vi "Process.vi"(8 "error in":errorcluster, 11 "Logger":refnum<class "Logger.PGSQL.lvclass">) -> (0 "error out":errorcluster, 3 "Logger out":refnum<class "Logger.PGSQL.lvclass">)   [LabVIEW 2019, in "Logger.PGSQL.lvlib" / "Logger.PGSQL.lvclass"]
doc: "---------------------------------------------------------------\nJKI State Machine Objects™\nhttp://jki.net/state-machine-objects/\nCopyright (C) 2005-2015, JKI <info@jki.net>\nALL RIGHTS RESERVED"
uses:
  Logger.PGSQL.lvclass
  C:/Program Files (x86)/National Instruments/LabVIEW 2019/vi.lib/JKI/JKI SMO/SMO/SMO.lvclass
  Logger.PGSQL.lvclass/Logger.PGSQL.ctl
  <vilib>/JKI/JKI SMO/SMO/SMO.lvclass/SMO.ctl
  <vilib>/JKI/JKI SMO/SMO/Private/ReftoDVR--SMO.vi
  <userlib>/LevyLab/LV-Data/LV-Data.PG/Private/INSERT Multivalue.vi
  <userlib>/LevyLab/Logger/Logger/Logger.lvclass
  <userlib>/LevyLab/Debug/Debug.lvlib
  <vilib>/JKI/JKI SMO/SMO/SMO.lvclass
  C:/Program Files (x86)/National Instruments/LabVIEW 2019/user.lib/LevyLab/Logger/Logger/Logger.lvclass
panel:
  out "Status":string
  out "State History":string
  out "Status Log":string
  out "Data":variant
  out "Address(es)":string
  # "DB Logger"
  # "For instructions on how to use the JKI State Machine Objects, examples and video tutorials, visit:\nhttp://jki.net/state-machine-objects/\n\nJKI State Machine Objects™\nhttp://jki.net/state-machine-objects/\nCopyright (C) 2005-2015, JKI <info@jki.net>\nALL RIGHTS RESERVED"
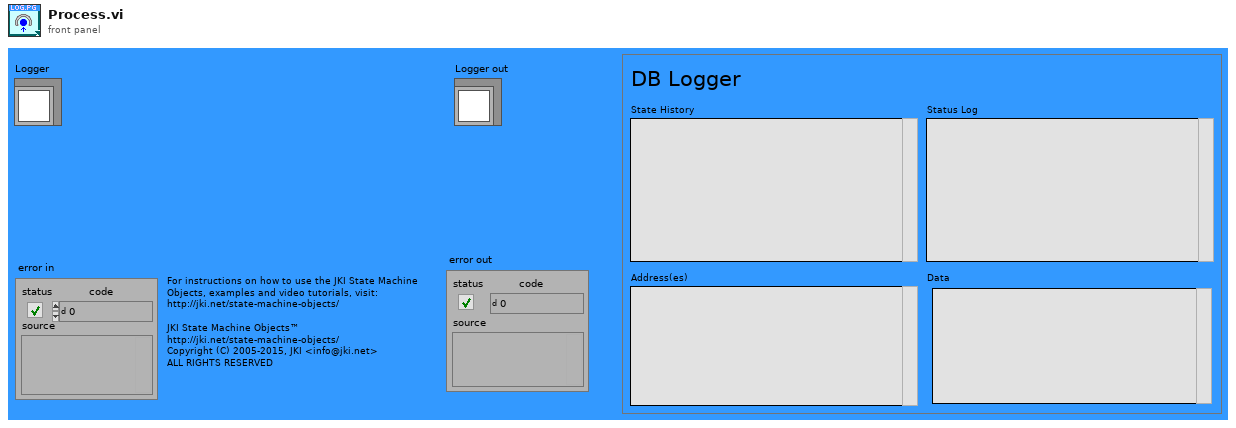
[diagram p1: front panel]
types:
  T1 = enum32{"invalid app kind", "Development System", "Run Time System", "Student Edition", "Embedded LabVIEW", "Evaluation", "Custom"}
  T2 = enum16{"unconfigured", "disconnected", "connected"}
  T3 = enum32{"Invalid", "Standard", "Closed", "Hidden", "Minimized", "Maximized"}
  T4 = cluster{"Core":cluster{"Current VI Reference":refnum<vi>, "Close Panel on Exit?":bool, "Last Error":cluster{"error":errorcluster, "previous state":string, "remaining states":string}, "Shutdown?":bool}, "SelfRef":refnum<class "Logger.PGSQL.lvclass">, "address":string, "data in":variant, "timestamps":timestamp[], "data out":variant, "Write Time":timestamp}
  T5 = cluster{"Current VI Reference":refnum<vi>, "Close Panel on Exit?":bool, "Last Error":cluster{"error":errorcluster, "previous state":string, "remaining states":string}, "Shutdown?":bool}
  T6 = typedef "Debug.lvlib/Attribute.Debug.lvclass/DebugBehavior.ctl" = enum16{"Normal", "Debug"}
  T7 = typedef "SMO.lvclass/Protected Events.ctl" = cluster{"StopProcesses":refnum<user-event>, "AbortProcesses":refnum<user-event>, "Config Changed":refnum<user-event>, "Dependency":refnum<user-event>}
  T8 = typedef "Logger.PGSQL.lvlib/Logger.PGSQL.lvclass/PrivateEvents--Cluster.ctl" = cluster{"Set Address":refnum<user-event>, "Write Variable":refnum<user-event>, "Read Variable":refnum<user-event>, "Write Variable Multiline":refnum<user-event>}
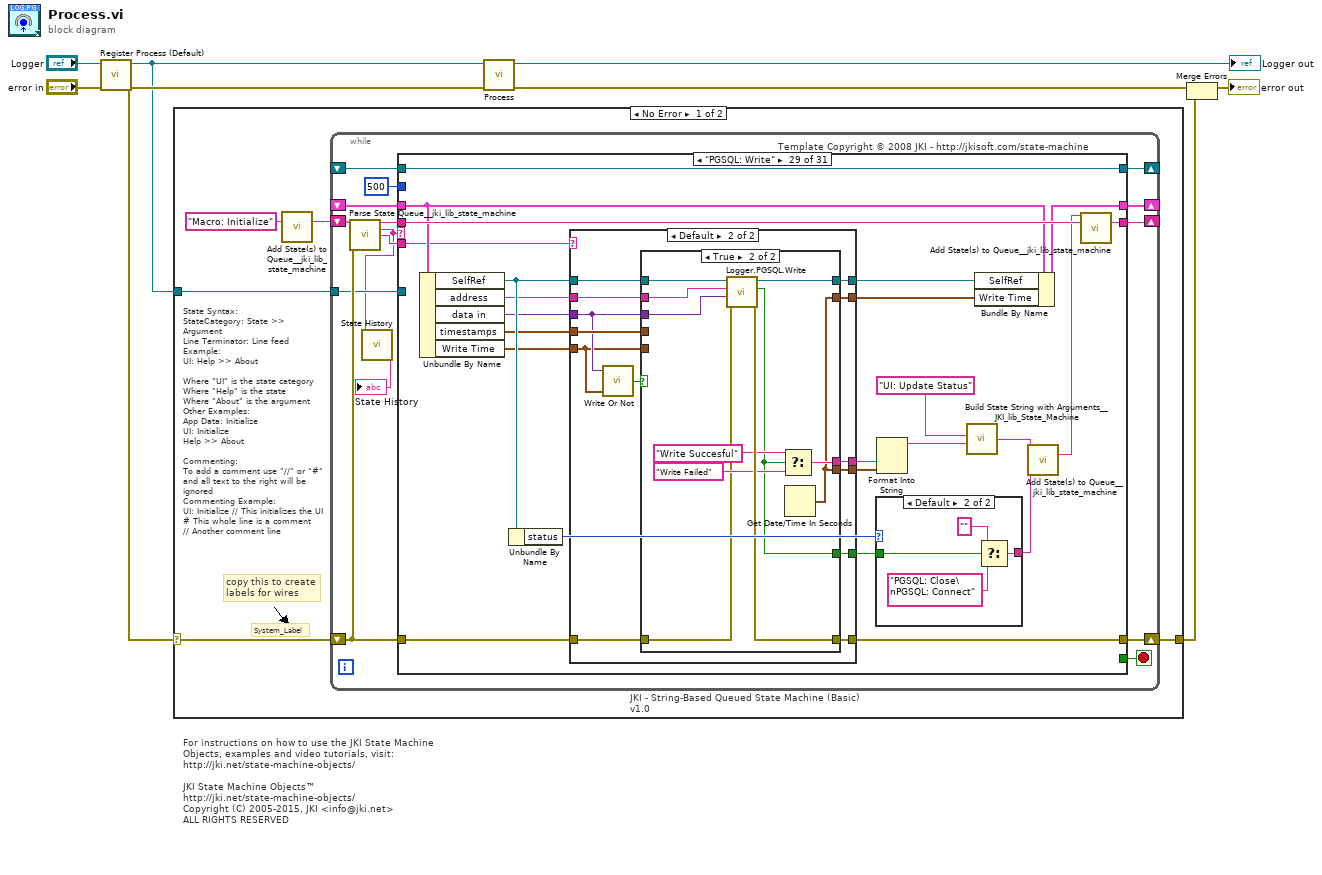
[diagram p0: block diagram]
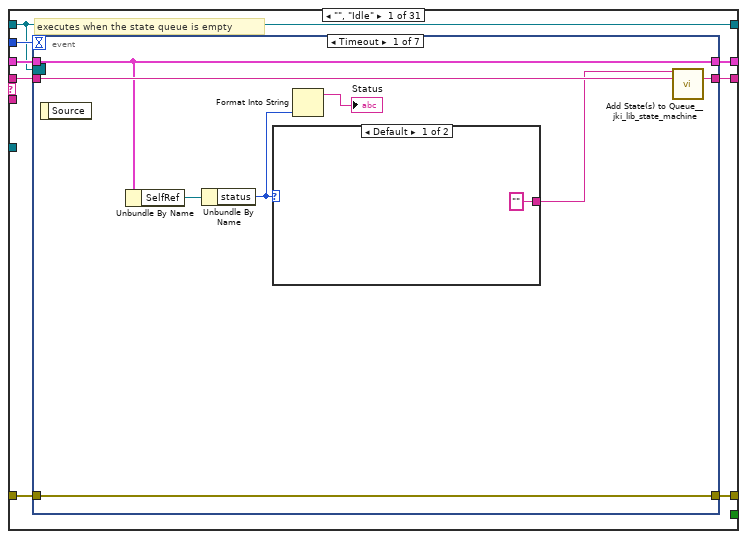
[diagram p2: hidden frame]
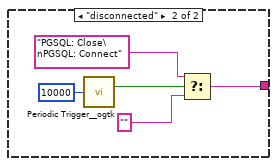
[diagram p3: hidden frame]
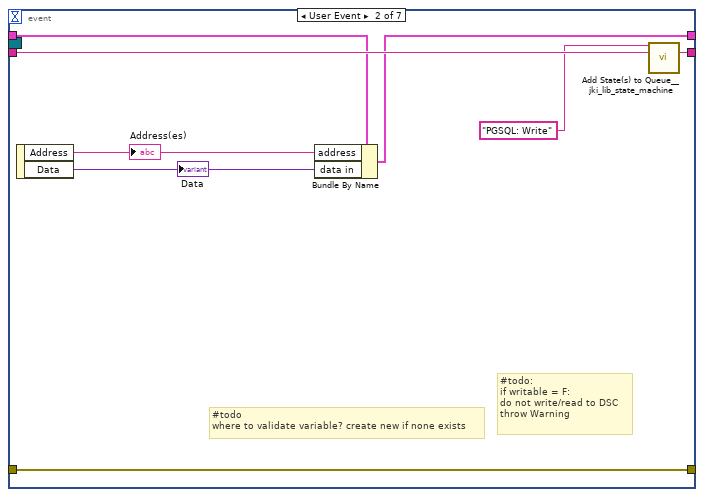
[diagram p4: hidden frame]
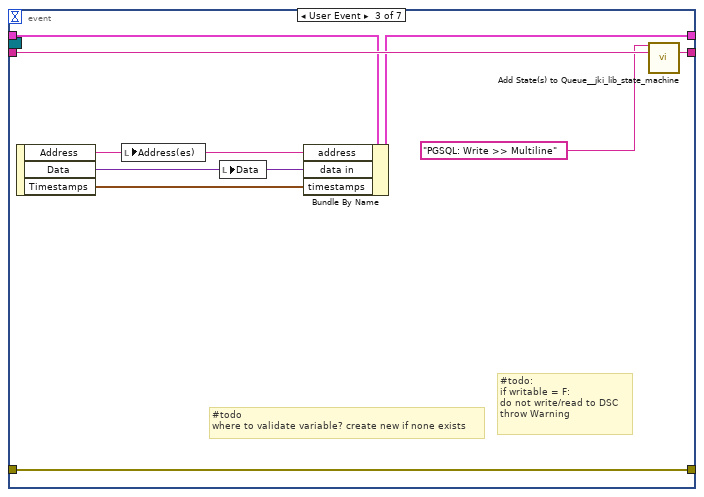
[diagram p5: hidden frame]
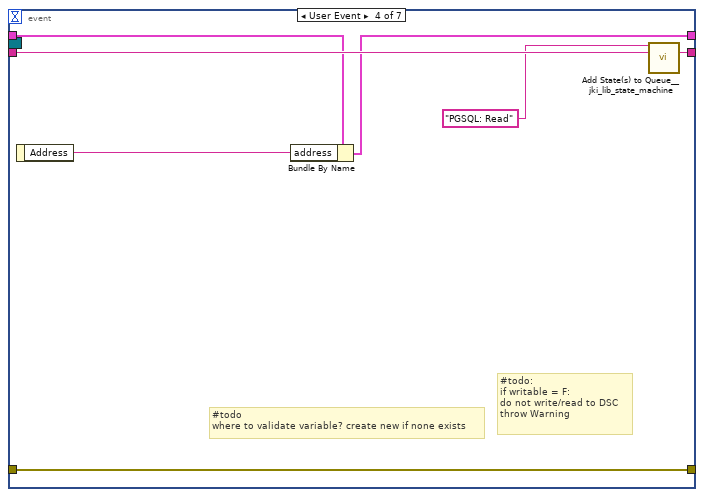
[diagram p6: hidden frame]
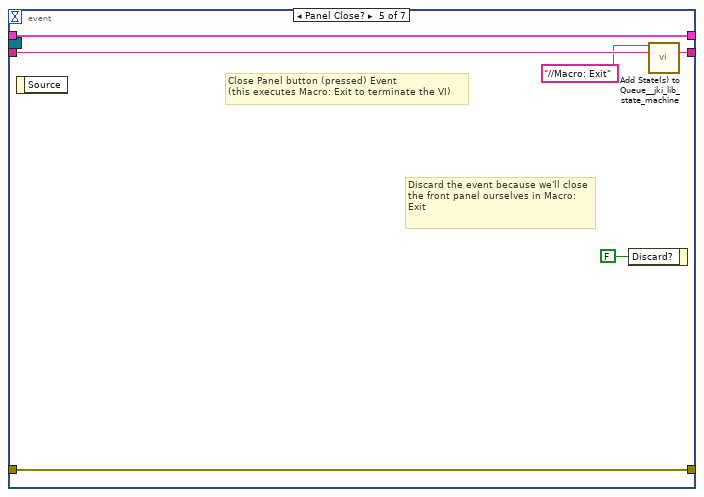
[diagram p7: hidden frame]
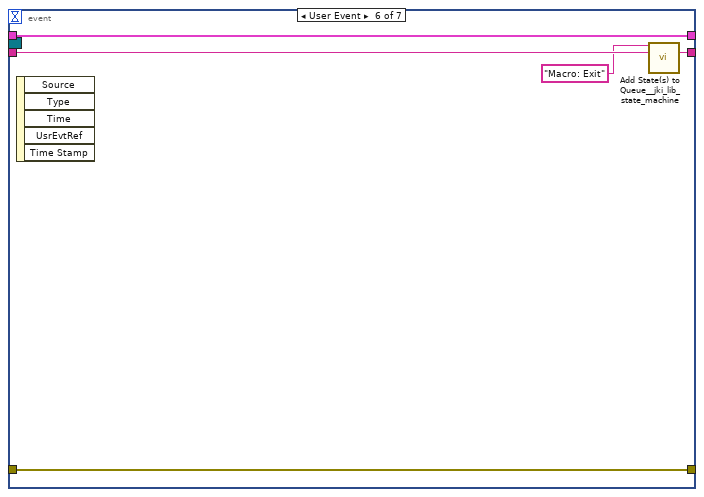
[diagram p8: hidden frame]
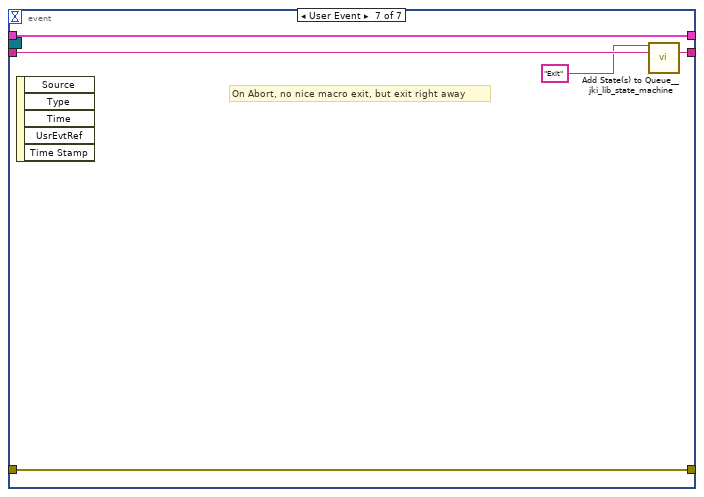
[diagram p9: hidden frame]
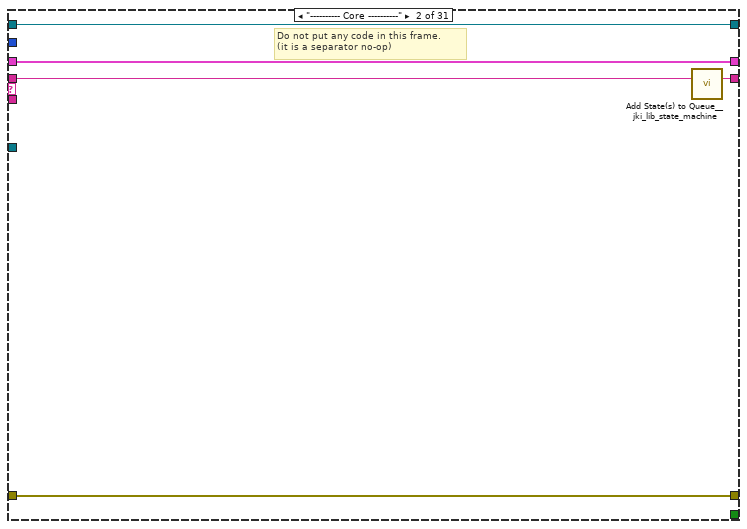
[diagram p10: hidden frame]
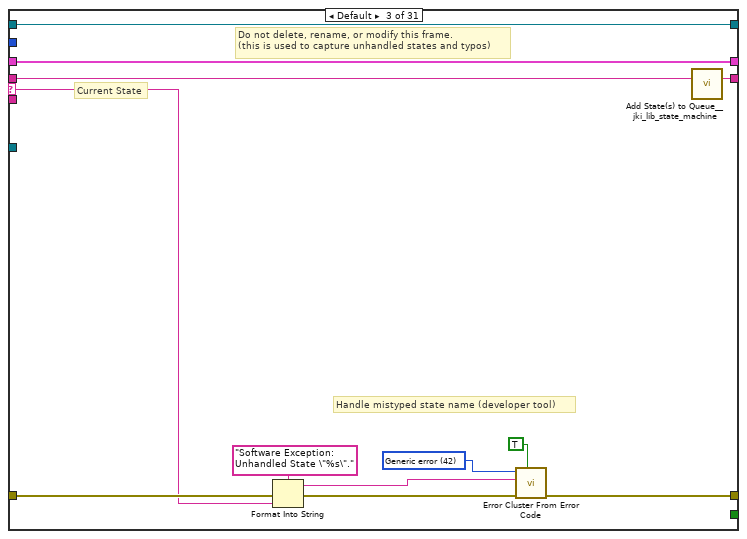
[diagram p11: hidden frame]
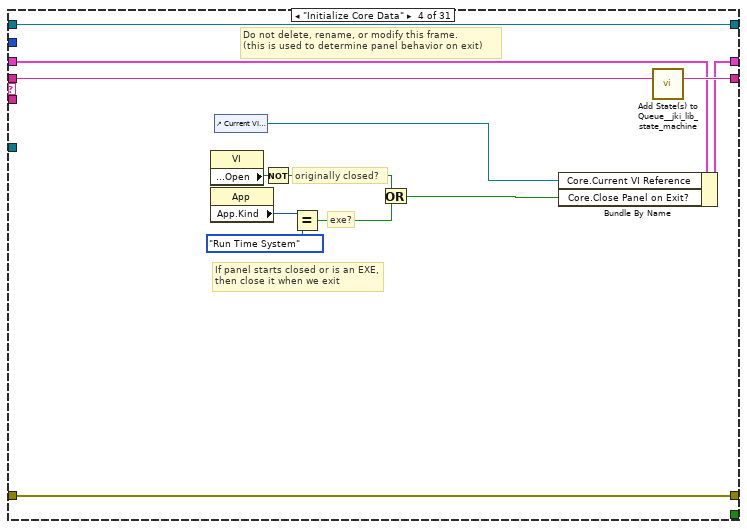
[diagram p12: hidden frame]
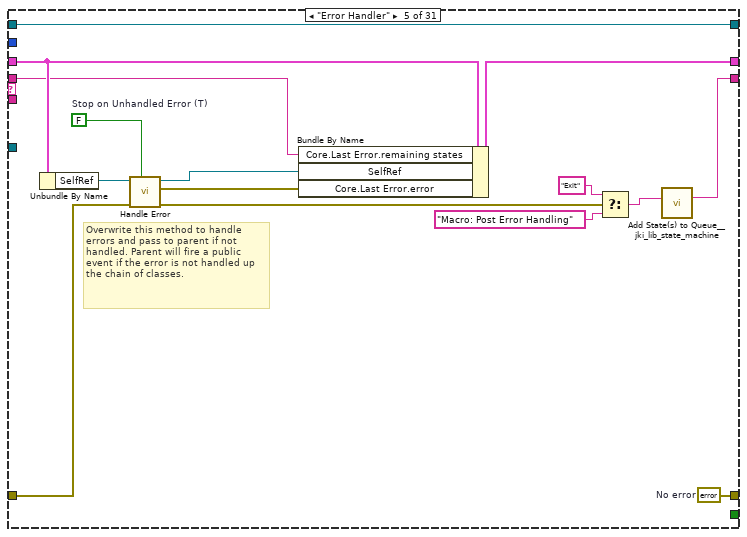
[diagram p13: hidden frame]
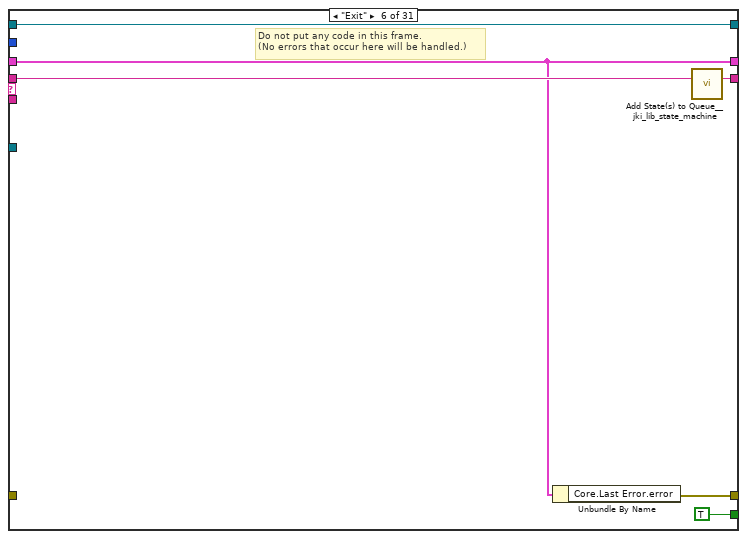
[diagram p14: hidden frame]
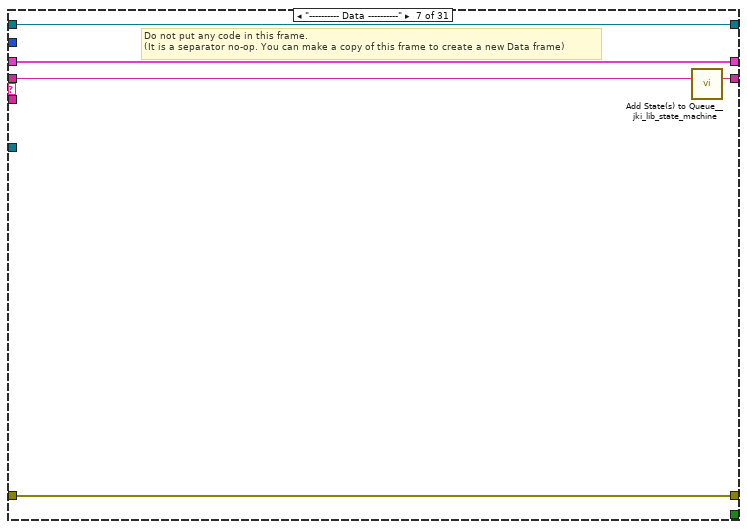
[diagram p15: hidden frame]
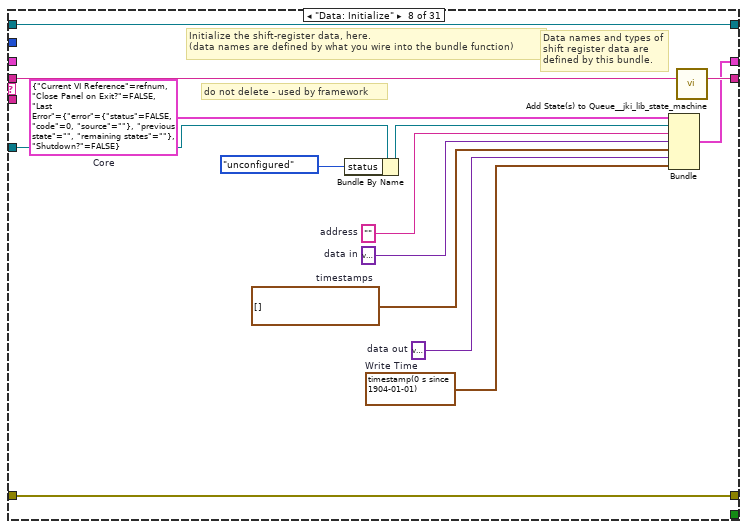
[diagram p16: hidden frame]
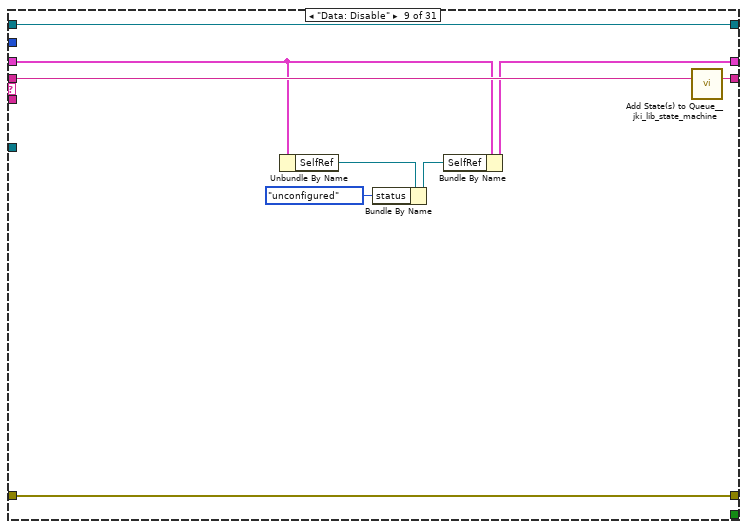
[diagram p17: hidden frame]
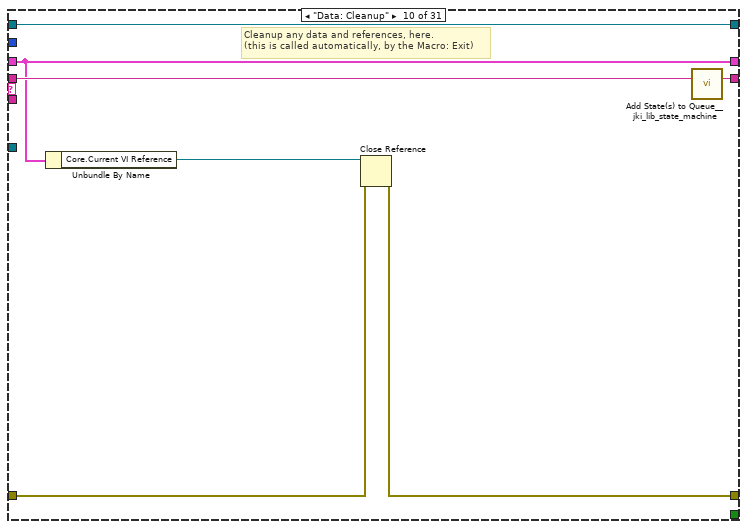
[diagram p18: hidden frame]
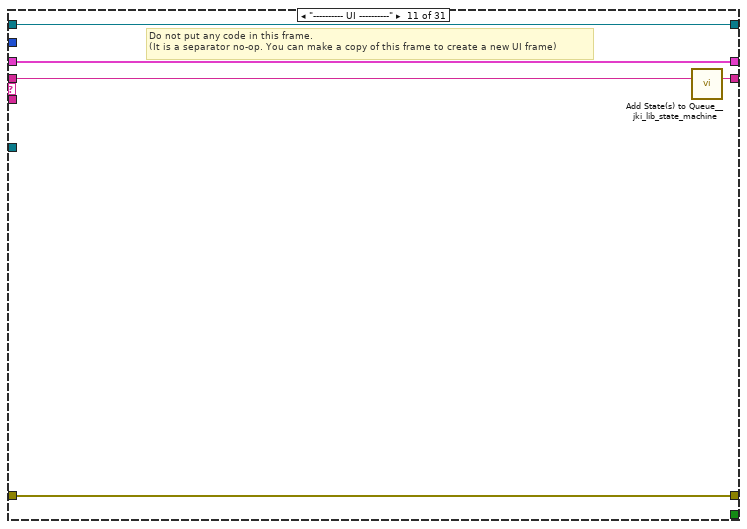
[diagram p19: hidden frame]
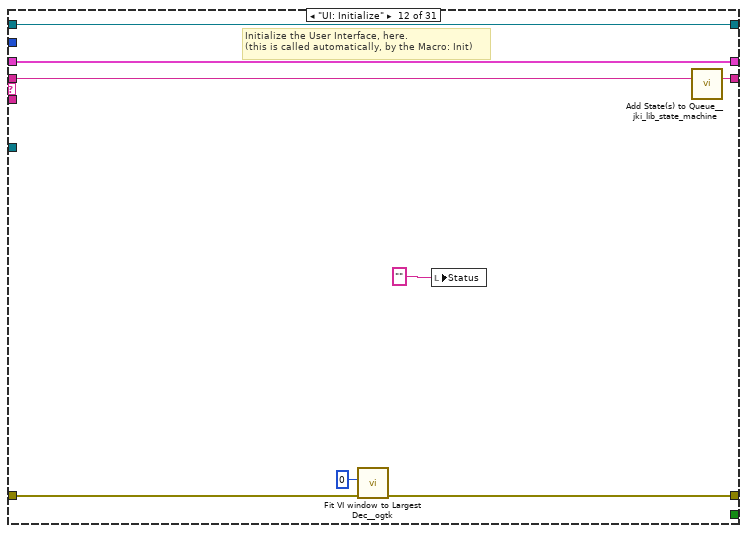
[diagram p20: hidden frame]
diagram:
  # "For instructions on how to use the JKI State Machine Objects, examples and video tutorials, visit:\nhttp://jki.net/state-machine-objects/\n\nJKI State Machine Objects™\nhttp://jki.net/state-machine-objects/\nCopyright (C) 2005-2015, JKI <info@jki.net>\nALL RIGHTS RESERVED"
  n1 = call <vilib>:"Register Process (Default).vi"("error in (no error)"="error in", "SMO"="Logger") -> ("error out"=w5:errorcluster, "SelfRef"=w4:refnum<class "Logger.PGSQL.lvclass">)  [unwired: 8 in]
  n2 = case shown="No Error" w5 {
    selector: w5 -> [w10 w477]
    tunnel: w4 -> [w11 _]
    tunnel: [w9 w477] -> w2
    frame No Error {
      # "State Syntax:\nStateCategory: State >> Argument\nLine Terminator: Line feed\nExample:\nUI: Help >> About\n\nWhere \"UI\" is the state category\nWhere \"Help\" is the state\nWhere \"About\" is the argument\nOther Examples:\nApp Data: Initialize\nUI: Initialize\nHelp >> About\n\nCommenting:\nTo add a comment use \"//\" or \"#\" and all text to the right will be ignored\nCommenting Example:\nUI: Initialize // This initializes the UI\n# This whole line is a comment\n// Another comment line"
      # "copy this to create labels for wires"
      # "System_Label"
      n3 = call <vilib>:"Add State(s) to Queue__jki_lib_state_machine.vi"("State(s) in (\"\")"="Macro: Initialize") -> ("States Out"=w13:string)  [unwired: 14 in]
      n4 = while "JKI - String-Based Queued State Machine (Basic) v1.0" {
        shift-right: [w23] -> _
        shift-left: _ -> [w22]
        shift-right: [w14] -> w9
        shift-left: w10 -> [w20]
        shift-right: [w25] -> _
        shift-left: w13 -> [w26]
        tunnel: w11 -> [w19]
        shift-right: [w18] -> _
        shift-left: _ -> [w17]
        stop <- w24 stop-if-true
        # "Template Copyright © 2008 JKI - http://jkisoft.com/state-machine"
        n5 = call <vilib>:"Parse State Queue__jki_lib_state_machine.vi"("State Queue"=w26, "Error In (no error)"=w20) -> ("Remaining States"=w28:string, "Current State"=w15:string, "Arguments"=w27:string)  [unwired: 11 in]
        n6 = call <userlib>:"State History.vi"("Current State"=w15) -> ("History"=→"State History":string)  [unwired: 10 in]
        n7 = case shown="\"PGSQL: Write\"" w15 {
          selector: w15 -> [_ _ w97 _ _ _ _ _ _ _ _ _ _ _ _ _ _ _ _ _ _ _ _ _ _ _ _ _ _ _ _]
          tunnel: w28 -> [w36 w95 w101 w120 w125 w141 w146 w160 w169 w176 w181 w189 w197 w204 w219 w227 w259 w270 w284 w302 w333 w338 w349 w354 w367 w373 w378 w387 w410 w467 w476]
          tunnel: w27 -> [_ _ _ _ _ _ _ _ _ _ _ _ w191 w198 w213 w221 _ _ _ _ _ _ _ _ _ _ _ _ w389 _ _]
          tunnel: w22 -> [w34 w92 w99 w111 w131 w137 w143 _ w164 w171 w178 w187 w194 w202 w216 w223 w256 w264 w272 w292 w318 w335 w346 w351 w365 w371 w376 w383 w406 w464 w473]
          tunnel: w20 -> [w32 w93 w102 w117 w133 _ w144 w151 w166 w173 w179 w184 w195 w200 w217 w225 w257 w260 w282 w300 w331 w336 w341 w352 w361 w369 w374 w380 w404 w462 w469]
          tunnel: [w35 w94 w100 w119 w123 w140 w145 w159 w168 w175 w180 w188 w196 w203 w218 w226 w258 w269 w283 w301 w332 w337 w348 w353 w366 w372 w377 w386 w409 w466 w475] -> w25
          tunnel: [_ _ _ _ _ TRUE _ _ _ _ _ _ _ _ _ _ _ _ _ _ _ _ _ _ _ _ _ _ _ _ _] -> w24
          tunnel: [w31 w92 w99 w118 w130 w137 w143 w158 w165 w171 w178 w187 w194 w202 w216 w223 w256 w264 w273 w293 w319 w335 w346 w351 w365 w371 w376 w384 w405 w464 w472] -> w23
          tunnel: 500 ("Timeout") -> [w30 _ _ _ _ _ _ _ _ _ _ _ _ _ _ _ _ _ _ _ _ _ _ _ _ _ _ _ _ _ _]
          tunnel: w19 -> [_ _ _ _ _ _ _ w148 _ _ _ _ _ _ _ _ _ _ _ _ _ _ _ _ _ _ _ _ _ _ _]
          tunnel: [w29 w91 w96 w108 w135 w138 w142 w157 w167 w170 w177 w186 w193 w201 w215 w220 w255 w268 w281 w299 w326 w334 w347 w350 w364 w370 w375 w385 w408 w465 w474] -> w18
          tunnel: w17 -> [w29 w91 w96 w108 w135 w138 w142 w157 w167 w170 w177 w186 w193 w201 w215 w220 w255 w268 w281 w299 w326 w334 w347 w350 _ w370 w375 w385 w408 w465 w474]
          tunnel: [w33 w93 w103 w117 w132 w136 w144 w151 w166 w172 w179 w185 w195 w199 w217 w224 w257 w260 w282 w300 w331 w336 w340 w352 w360 w369 w374 w379 w407 w461 w468] -> w14
          frame "", "Idle" {
            # "executes when the state queue is empty"
            n8 = event shown="[0] Timeout" {
              selector: w29 -> [_ _ _ _ _ _ _]
              dyn-events: _ -> [_ _ _ _ _ _ _]
              timeout: w30 -> [_ _ _ _ _ _ _]
              tunnel: w36 -> [w44 w58 w67 w74 w80 w85 w90]
              tunnel: [w43 w57 w66 w73 w79 w84 w89] -> w35
              tunnel: w34 -> [w41 w55 w64 w71 w77 w82 w87]
              tunnel: [w42 w56 w65 w72 w78 w83 w88] -> w33
              tunnel: w32 -> [w42 w56 w65 w72 w78 w83 w88]
              tunnel: [w41 w52 w60 w69 w77 w82 w87] -> w31
              event Timeout {
                n9 = event-data() -> ()  [unwired: 1 in, 1 out]
                n10 = Unbundle By Name(w41) -> ("SelfRef"=w40:refnum<class "Logger.PGSQL.lvclass">)
                n11 = Unbundle By Name(w40) -> ("status"=w38:T2)
                n12 = case shown="Default" w38 {
                  tunnel: ["" w48] -> w39
                  frame Default {
                  }
                  frame "disconnected" {
                    n13 = call <userlib>:"Periodic Trigger__ogtk.vi"("time (ms)"=u32 10000) -> ("Triggered"=w50:bool)  [unwired: 12 in, 2 out]
                    n14 = Select(t="PGSQL: Close\nPGSQL: Connect", s=w50, f="") -> (s? t:f=w48:string)
                  }
                }
                n15 = Format Into String(w38) -> (resulting string=→"Status":string)  [unwired: 3 in, 1 out]
                n16 = call <vilib>:"Add State(s) to Queue__jki_lib_state_machine.vi"("State(s) in Front (\"\")"=w39, "State(s) in (\"\")"=w44) -> ("States Out"=w43:string)  [unwired: 13 in]
              }
              event User Event {
                # "#todo:\nif writable = F:\ndo not write/read to DSC\nthrow Warning"
                # "#todo\nwhere to validate variable? create new if none exists"
                n17 = event-data() -> ("Address"=w53:string, "Data"=w54:variant)  [unwired: 1 in]
                "Address(es)" <- w53
                "Data" <- w54
                n18 = Bundle By Name(cluster=w55, "address"=w53, "data in"=w54) -> (w52:T4)
                n19 = call <vilib>:"Add State(s) to Queue__jki_lib_state_machine.vi"("State(s) in Front (\"\")"="PGSQL: Write" ("State(s) in Front (\"\")"), "State(s) in (\"\")"=w58) -> ("States Out"=w57:string)  [unwired: 13 in]
              }
              event User Event {
                # "#todo:\nif writable = F:\ndo not write/read to DSC\nthrow Warning"
                # "#todo\nwhere to validate variable? create new if none exists"
                n20 = event-data() -> ("Address"=w63:string, "Data"=w62:variant, "Timestamps"=w61:timestamp[])  [unwired: 1 in]
                n21 = local write "Address(es)"(w63) -> ()
                n22 = local write "Data"(w62) -> ()
                n23 = Bundle By Name(cluster=w64, "address"=w63, "data in"=w62, "timestamps"=w61) -> (w60:T4)
                n24 = call <vilib>:"Add State(s) to Queue__jki_lib_state_machine.vi"("State(s) in Front (\"\")"="PGSQL: Write >> Multiline" ("State(s) in Front (\"\")"), "State(s) in (\"\")"=w67) -> ("States Out"=w66:string)  [unwired: 13 in]
              }
              event User Event {
                # "#todo:\nif writable = F:\ndo not write/read to DSC\nthrow Warning"
                # "#todo\nwhere to validate variable? create new if none exists"
                n25 = event-data() -> ("Address"=w70:string)  [unwired: 1 in]
                n26 = Bundle By Name(cluster=w71, "address"=w70) -> (w69:T4)
                n27 = call <vilib>:"Add State(s) to Queue__jki_lib_state_machine.vi"("State(s) in Front (\"\")"="PGSQL: Read" ("State(s) in Front (\"\")"), "State(s) in (\"\")"=w74) -> ("States Out"=w73:string)  [unwired: 13 in]
              }
              event Panel Close? {
                # "Discard the event because we'll close the front panel ourselves in Macro: Exit"
                # "Close Panel button (pressed) Event\n(this executes Macro: Exit to terminate the VI)"
                n28 = event-data() -> ()  [unwired: 1 in, 1 out]
                n29 = event-data("Discard?"=FALSE) -> ()  [unwired: 1 in, 1 out]
                n30 = call <vilib>:"Add State(s) to Queue__jki_lib_state_machine.vi"("State(s) in Front (\"\")"="//Macro: Exit", "State(s) in (\"\")"=w80) -> ("States Out"=w79:string)  [unwired: 13 in]
              }
              event User Event {
                n31 = event-data() -> ()  [unwired: 1 in, 5 out]
                n32 = call <vilib>:"Add State(s) to Queue__jki_lib_state_machine.vi"("State(s) in Front (\"\")"="Macro: Exit", "State(s) in (\"\")"=w85) -> ("States Out"=w84:string)  [unwired: 13 in]
              }
              event User Event {
                # "On Abort, no nice macro exit, but exit right away"
                n33 = event-data() -> ()  [unwired: 1 in, 5 out]
                n34 = call <vilib>:"Add State(s) to Queue__jki_lib_state_machine.vi"("State(s) in Front (\"\")"="Exit", "State(s) in (\"\")"=w90) -> ("States Out"=w89:string)  [unwired: 13 in]
              }
            }
          }
          frame "---------- Core ----------" {
            # "Do not put any code in this frame.\n(it is a separator no-op)"
            n35 = call <vilib>:"Add State(s) to Queue__jki_lib_state_machine.vi"("State(s) in (\"\")"=w95) -> ("States Out"=w94:string)  [unwired: 14 in]
          }
          frame Default {
            w106 = 42 items=["No error", "Argument error", "Memory is full", "Out of zone", "End of file", "File already open", "Generic file I/O error", "File not found", "File permission error", "Disk is full", "Duplicate path", "Too many files open", "System feature not enabled", "Resource file not found", "Cannot add resource", "Resource not found", "Image not found", "Image memory error", "Pen does not exist", "Config type invalid", "Config token not found", "Config parse error", "Config memory error", "Bad external code format", "Bad external code offset", "External code not present", "Null window", "Destroy window error", "Null menu", "Print aborted", "Bad print record", "Print driver error", "Windows error during printing", "Memory error during printing", "Print dialog error", "Generic print error", "Invalid device refnum", "Device not found", "Device parameter error", "Device unit error", "Cannot open device", "Device call aborted", "Generic error", "Cancelled by user", "Object ID too low", "Object ID too high", "Object not in heap", "Unknown heap", "Unknown object (invalid DefProc)", "Unknown object (DefProc not in table)", "Message out of range", "Invalid (null) method", "Unknown message", "Manager call not supported", "Bad address", "Network operation in progress", "Network operation timed out", "Connection is busy", "Network attribute not supported", "Network error", "Address in use", "System out of memory", "Connection aborted", "Connection refused", "Not connected", "Already connected", "Connection closed", "Initialization error (interapplication manager)", "Bad occurrence", "Wait on unbound occurrence handler", "Occurrence queue overflow", "Datalog type conflict", "Unused", "Unrecognized type (interapplication manager)", "Memory corrupt", "Failed to make temporary DLL", "Old CIN version", "Drag socket not found", "Failed to load drop-object", "Failed to register OLE object", "Failed to release OLE object", "Format specifier type mismatch", "Unknown format specifier", "Too few format specifiers", "Too many format specifiers", "Scan failed", "Newer CIN version", "Error converting to variant", "Runtime menu error", "Password tampered", "Variant attribute not found", "Incompatible variant data type", "Event data is not available", "Event Store is not present", "Occurrence is not found", "Event Queue is not created", "Event info is not available", "Refnum passed is NULL", "Error retrieving Class GUID", "Error retrieving CoClass GUID", "Error retrieving TypeLib GUID.", "Bad built application magic bytes.", "Specific driver is different from the specific driver associated with the Logical Name.", "There is no session opened to the class driver.", "Max Error", "MAX - Error with config objects", "MAX - Error loading configuration", "MAX - Group not supported"]
            # "Current State"
            # "Do not delete, rename, or modify this frame.\n(this is used to capture unhandled states and typos)"
            # "Handle mistyped state name (developer tool)"
            n36 = Format Into String(format string="Software Exception: Unhandled State \"%s\"." ("message"), error in=w102, w97) -> (resulting string=w105:string, error out=w104:errorcluster)  [unwired: 1 in]
            n37 = call <vilib>:"Error Cluster From Error Code.vi"("show call chain? (False)"=TRUE, "error in (no error)"=w104, "error message (\"\")"=w105, "error code (0)"=w106) -> ("error out"=w103:errorcluster)  [unwired: 5 in]
            n38 = call <vilib>:"Add State(s) to Queue__jki_lib_state_machine.vi"("State(s) in (\"\")"=w101) -> ("States Out"=w100:string)  [unwired: 14 in]
          }
          frame "Initialize Core Data" {
            # "Do not delete, rename, or modify this frame.\n(this is used to determine panel behavior on exit)"
            # "originally closed?"
            # "exe?"
            # "If panel starts closed or is an EXE, then close it when we exit"
            n39 = property class="VI"() -> ("Front Panel.Open"=w116:bool)  [unwired: 2 in, 2 out]
            n40 = property class="App"() -> ("App.Kind"=w115:T1)  [unwired: 2 in, 2 out]
            n41 = control-ref of="Current VI Reference"() -> (w109:refnum<vi>)
            n42 = Not(x=w116) -> (.not. x?=w113:bool)
            n43 = Equal?(x=w115, y=T1."Run Time System" ("Application:Kind")) -> (x = y?=w112:bool)
            n44 = Or(x=w113, y=w112) -> (x .or. y?=w110:bool)
            n45 = Bundle By Name(cluster=w111, "Core.Current VI Reference"=w109, "Core.Close Panel on Exit?"=w110) -> (w118:T4)
            n46 = call <vilib>:"Add State(s) to Queue__jki_lib_state_machine.vi"("State(s) in (\"\")"=w120) -> ("States Out"=w119:string)  [unwired: 14 in]
          }
          frame "Error Handler" {
            w127 = FALSE  # Stop on Unhandled Error (T)
            w132 = errorcluster {"status"=FALSE, "code"=0, "source"=""}  # No error
            # "Overwrite this method to handle errors and pass to parent if not handled. Parent will fire a public event if the error is not handled up the chain of classes."
            n47 = Unbundle By Name(w131) -> ("SelfRef"=w134:refnum<class "Logger.PGSQL.lvclass">)
            n48 = call-dynamic "Handle Error.vi"("Stop on Unhandled Error (T)"=w127, "error in"=w133, "Logger.PGSQL"=w134) -> ("handling error"=w128:errorcluster, "Unhandled error"=w126:errorcluster, "Logger.PGSQL out"=w121:refnum<class "Logger.PGSQL.lvclass">)  [unwired: 6 in]
            n49 = Bundle By Name(cluster=w131, "Core.Last Error.remaining states"=w125, "SelfRef"=w121, "Core.Last Error.error"=w126) -> (w130:T4)
            n50 = Select(t="Exit", s=w128, f="Macro: Post Error Handling") -> (s? t:f=w122:string)
            n51 = call <vilib>:"Add State(s) to Queue__jki_lib_state_machine.vi"("State(s) in (\"\")"=w122) -> ("States Out"=w123:string)  [unwired: 14 in]
          }
          frame "Exit" {
            # "Do not put any code in this frame.\n(No errors that occur here will be handled.)"
            n52 = Unbundle By Name(w137) -> ("Core.Last Error.error"=w136:errorcluster)
            n53 = call <vilib>:"Add State(s) to Queue__jki_lib_state_machine.vi"("State(s) in (\"\")"=w141) -> ("States Out"=w140:string)  [unwired: 14 in]
          }
          frame "---------- Data ----------" {
            # "Do not put any code in this frame.\n(It is a separator no-op. You can make a copy of this frame to create a new Data frame)"
            n54 = call <vilib>:"Add State(s) to Queue__jki_lib_state_machine.vi"("State(s) in (\"\")"=w146) -> ("States Out"=w145:string)  [unwired: 14 in]
          }
          frame "Data: Initialize" {
            w150 = timestamp[] []  # timestamps
            w152 = timestamp(0 s since 1904-01-01)  # Write Time
            w153 = variant  # data out
            w154 = variant  # data in
            w155 = ""  # address
            w156 = T5 {"Current VI Reference"=refnum, "Close Panel on Exit?"=FALSE, "Last Error"={"error"={"status"=FALSE, "code"=0, "source"=""}, "previous state"="", "remaining states"=""}, "Shutdown?"=FALSE}  # Core
            # "do not delete - used by framework"
            # "Data names and types of shift register data are defined by this bundle."
            # "Initialize the shift-register data, here.\n(data names are defined by what you wire into the bundle function)"
            n55 = Bundle By Name(cluster=w148, "status"=T2."unconfigured") -> (w149:refnum<class "Logger.PGSQL.lvclass">)
            n56 = Bundle("Core"=w156, "SelfRef"=w149, "address"=w155, "data in"=w154, "timestamps"=w150, "data out"=w153, "Write Time"=w152) -> (w158:T4)  [unwired: 1 in]
            n57 = call <vilib>:"Add State(s) to Queue__jki_lib_state_machine.vi"("State(s) in (\"\")"=w160) -> ("States Out"=w159:string)  [unwired: 14 in]
          }
          frame "Data: Disable" {
            n58 = Unbundle By Name(w164) -> ("SelfRef"=w163:refnum<class "Logger.PGSQL.lvclass">)
            n59 = Bundle By Name(cluster=w163, "status"=T2."unconfigured") -> (w162:refnum<class "Logger.PGSQL.lvclass">)
            n60 = Bundle By Name(cluster=w164, "SelfRef"=w162) -> (w165:T4)
            n61 = call <vilib>:"Add State(s) to Queue__jki_lib_state_machine.vi"("State(s) in (\"\")"=w169) -> ("States Out"=w168:string)  [unwired: 14 in]
          }
          frame "Data: Cleanup" {
            # "Cleanup any data and references, here.\n(this is called automatically, by the Macro: Exit)"
            n62 = Unbundle By Name(w171) -> ("Core.Current VI Reference"=w174:refnum<vi>)
            n63 = Close Reference(reference=w174, error in (no error)=w173) -> (error out=w172:errorcluster)
            n64 = call <vilib>:"Add State(s) to Queue__jki_lib_state_machine.vi"("State(s) in (\"\")"=w176) -> ("States Out"=w175:string)  [unwired: 14 in]
          }
          frame "---------- UI ----------" {
            # "Do not put any code in this frame.\n(It is a separator no-op. You can make a copy of this frame to create a new UI frame)"
            n65 = call <vilib>:"Add State(s) to Queue__jki_lib_state_machine.vi"("State(s) in (\"\")"=w181) -> ("States Out"=w180:string)  [unwired: 14 in]
          }
          frame "UI: Initialize" {
            # "Initialize the User Interface, here.\n(this is called automatically, by the Macro: Init)"
            n66 = call <userlib>:"Fit VI window to Largest Dec__ogtk.vi"("error in (no error)"=w184, "border spacing (2 px)"=0) -> ("error out"=w185:errorcluster)  [unwired: 4 in, 1 out]
            n67 = local write "Status"("" ("Status")) -> ()
            n68 = call <vilib>:"Add State(s) to Queue__jki_lib_state_machine.vi"("State(s) in (\"\")"=w189) -> ("States Out"=w188:string)  [unwired: 14 in]
          }
          frame "UI: Wait" {
            n69 = Scan From String(input string=w191, default 1=u32 0) -> (output 1=w190:u32)  [unwired: 3 in, 3 out]
            n70 = Wait (ms)(milliseconds to wait=w190) -> ()  [unwired: 1 out]
            n71 = call <vilib>:"Add State(s) to Queue__jki_lib_state_machine.vi"("State(s) in (\"\")"=w197) -> ("States Out"=w196:string)  [unwired: 14 in]
          }
          frame "UI: Cursor Set" {
            # "Argument"
            # "Initialize the User Interface, here.\n(this is called automatically, by the Macro: Init)"
            n72 = disable-structure shown="Default" {
              disable-tunnel: w200 -> [w205 w208]
              disable-tunnel: [w205 w207] -> w199
              disable-tunnel: w198 -> [_ w206]
              frame condition #0 {
              }
              frame condition #1 (active) {
                n73 = case shown="\"Idle\", Default" w206 {
                  tunnel: w208 -> [w210 w212]
                  tunnel: [w209 w211] -> w207
                  frame "Idle", Default {
                    n74 = call <vilib>:"Unset Busy.vi"("error in (no error)"=w210) -> ("error out"=w209:errorcluster)  [unwired: 10 in]
                  }
                  frame "Busy" {
                    n75 = call <vilib>:"Set Busy.vi"("error in (no error)"=w212) -> ("error out"=w211:errorcluster)  [unwired: 9 in, 1 out]
                  }
                }
              }
            }
            n76 = call <vilib>:"Add State(s) to Queue__jki_lib_state_machine.vi"("State(s) in (\"\")"=w204) -> ("States Out"=w203:string)  [unwired: 14 in]
          }
          frame "UI: Update Status" {
            # "Do not put any code in this frame.\n(It is a separator no-op. You can make a copy of this frame to create a new UI frame)"
            n77 = call <userlib>:"State History.vi"("Current State"=w213) -> ("History"=→"Status Log":string)  [unwired: 10 in]
            n78 = call <vilib>:"Add State(s) to Queue__jki_lib_state_machine.vi"("State(s) in (\"\")"=w219) -> ("States Out"=w218:string)  [unwired: 14 in]
          }
          frame "UI: Front Panel State" {
            # "Argument"
            # "Set Front Panel Open or Closed\n(Usage: \"UI: Front Panel State >> Open|Close\")"
            n79 = Unbundle By Name(w223) -> ("Core.Current VI Reference"=w222:refnum<vi>)
            n80 = disable-structure shown="Default" {
              disable-tunnel: w225 -> [w231 w254]
              disable-tunnel: [w230 w254] -> w224
              disable-tunnel: w222 -> [w229 _]
              disable-tunnel: w221 -> [w228 _]
              frame condition #0 (active) {
                n81 = case shown="\"Close\"" w228 {
                  tunnel: w231 -> [w235 w248]
                  tunnel: [w237 w249] -> w230
                  tunnel: w229 -> [w236 w246]
                  frame "Open", Default {
                    n82 = property class="VI"(reference=w236, error in=w235) -> (reference out=w233:refnum<vi>, error out=w234:errorcluster, "FP.State"=w232:T3)
                    n83 = case shown="\"Closed\"" w232 {
                      tunnel: [w240 w243] -> w237
                      tunnel: w234 -> [w239 w243]
                      tunnel: w233 -> [w238 _]
                      frame "Closed" {
                        n84 = invoke class="VI" method="FP.Open"(reference=w238, error in=w239, "Activate"=TRUE, "State"=T3."Standard") -> (error out=w240:errorcluster)  [unwired: 1 in, 4 out]
                      }
                      frame Default {
                      }
                    }
                  }
                  frame "Close" {
                    n85 = property class="VI"(reference=w246, error in=w248) -> (reference out=w245:refnum<vi>, error out=w247:errorcluster, "FP.State"=w244:T3)
                    n86 = case shown="Default" w244 {
                      tunnel: [w250 w253] -> w249
                      tunnel: w247 -> [w250 w252]
                      tunnel: w245 -> [_ w251]
                      frame "Invalid", "Closed" {
                      }
                      frame Default {
                        n87 = invoke class="VI" method="FP.Close"(reference=w251, error in=w252) -> (error out=w253:errorcluster)  [unwired: 1 in, 2 out]
                      }
                    }
                  }
                }
              }
              frame condition #1 {
              }
            }
            n88 = call <vilib>:"Add State(s) to Queue__jki_lib_state_machine.vi"("State(s) in (\"\")"=w227) -> ("States Out"=w226:string)  [unwired: 14 in]
          }
          frame "---------- Macro ----------" {
            # "Do not put any code in this frame.\n(It is a separator no-op. You can make a copy of this frame to create a new Macro frame)"
            n89 = call <vilib>:"Add State(s) to Queue__jki_lib_state_machine.vi"("State(s) in (\"\")"=w259) -> ("States Out"=w258:string)  [unwired: 14 in]
          }
          frame "Macro: Initialize" {
            # "Initialization Macro\n(This is called once, when the VI starts)"
            n90 = call <vilib>:"Add State(s) to Queue__jki_lib_state_machine.vi"("State(s) in Front (\"\")"="UI: Initialize", "State(s) in (\"\")"="UI: Front Panel State >> Close\nMacro: Debug\nPGSQL: Connect") -> ("States Out"=w262:string)  [unwired: 13 in]
            n91 = call <vilib>:"Add State(s) to Queue__jki_lib_state_machine.vi"("State(s) in Front (\"\")"="Data: Initialize\nInitialize Core Data\nEvents: Register", "State(s) in (\"\")"="Process: Sync", "State(s) at Back (\"\")"=w262) -> ("States Out"=w266:string)  [unwired: 12 in]
            n92 = call <vilib>:"Add State(s) to Queue__jki_lib_state_machine.vi"("State(s) in Front (\"\")"=w266, "State(s) in (\"\")"=w270) -> ("States Out"=w269:string)  [unwired: 13 in]
          }
          frame "Macro: Debug" {
            # "exe?"
            # "If pane is an EXE, then close it when we exit"
            # "Macro: Debug\n(get debug behavior, determine UI and determine shutdown behavior)"
            n93 = Unbundle By Name(w272) -> ("Core.Close Panel on Exit?"=w275:bool, "SelfRef"=w280:refnum<class "Logger.PGSQL.lvclass">)
            n94 = property class="App"() -> ("App.Kind"=w278:T1)  [unwired: 2 in, 2 out]
            n95 = Equal?(x=w278, y=T1."Run Time System" ("Application:Kind")) -> (x = y?=w274:bool)
            n96 = call <userlib>:"Get Debug Mode.vi"("SMO"=w280) -> ("Behavior"=w279:T6)  [unwired: 8 in, 2 out]
            n97 = case shown="\"Debug\"" w279 {
              tunnel: [_ "UI: Front Panel State >> Open\nUI: Wait >> 1000"] -> w271
              tunnel: [w285 w286] -> w276
              tunnel: w275 -> [w285 _]
              tunnel: w274 -> [_ w288]
              frame "Normal", Default {
                # "respect core.close"
              }
              frame "Debug" {
                # "keep panel open\nunless exe"
                n98 = Or(x=w288, y=FALSE) -> (x .or. y?=w286:bool)
              }
            }
            n99 = Bundle By Name(cluster=w272, "Core.Close Panel on Exit?"=w276) -> (w273:T4)
            n100 = call <vilib>:"Add State(s) to Queue__jki_lib_state_machine.vi"("State(s) in Front (\"\")"=w271, "State(s) in (\"\")"=w284) -> ("States Out"=w283:string)  [unwired: 13 in]
          }
          frame "Macro: Post Error Handling" {
            # "Clear Last Error?"
            n101 = Unbundle By Name(w292) -> ("SelfRef"=w290:refnum<class "Logger.PGSQL.lvclass">, "Core.Last Error.remaining states"=w294:string, "Core.Shutdown?"=w295:bool)
            n102 = Unbundle By Name(w292) -> ("Core.Last Error.error"=w298:errorcluster)
            n103 = case shown="False" FALSE {
              tunnel: w298 -> [w317 _]
              tunnel: [w317 _] -> w297
              frame False {
              }
              frame True {
              }
            }
            n104 = case shown="False" w295 {
              tunnel: w294 -> [w303 w316]
              tunnel: [w305 w315] -> w291
              tunnel: w290 -> [w307 _]
              frame False {
                # "These are the remaining states (at the moment the error occured). States can be altered according to business logic."
                # "NOT SHUTTING DOWN"
                n105 = Unbundle By Name(w307) -> ("status"=w304:T2, "retry counter"=w306:i32)
                n106 = case shown="\"unconfigured\"" w304 {
                  tunnel: w306 -> [_ w314]
                  tunnel: [w308 w309] -> w305
                  tunnel: w303 -> [w308 _]
                  frame Default {
                  }
                  frame "unconfigured" {
                    n107 = Less?(x=w314, y=2) -> (x < y?=w312:bool)
                    n108 = Select(t="UI: Wait >> 2000\nPGSQL: Connect", s=w312, f="Data: Disable") -> (s? t:f=w309:string)
                  }
                }
              }
              frame True {
                # "Developer can decide to alter the states but should be aware that during the shutdown process, there are certain states that must be run for the SMO to properly shut itself (and this process) down. As such, one can add states to perform additional clean-ups, but should append the remaining state to be executed."
                # "SHUTTING DOWN"
                n109 = call <vilib>:"Add State(s) to Queue__jki_lib_state_machine.vi"("State(s) in (\"\")"=w316) -> ("States Out"=w315:string)  [unwired: 14 in]
              }
            }
            n110 = Bundle By Name(cluster=w292, "Core.Last Error.error"=w297) -> (w293:T4)
            n111 = call <vilib>:"Add State(s) to Queue__jki_lib_state_machine.vi"("State(s) in Front (\"\")"=w291, "State(s) in (\"\")"=w302) -> ("States Out"=w301:string)  [unwired: 13 in]
          }
          frame "Macro: Exit" {
            # "Exit Macro\n(This is called once, when the VI exits)"
            n112 = Unbundle By Name(w318) -> ("Core.Close Panel on Exit?"=w330:bool)
            n113 = Bundle By Name(cluster=w318, "Core.Shutdown?"=TRUE) -> (w319:T4)
            n114 = Select(t="UI: Front Panel State >> Close", s=w330, f="") -> (s? t:f=w328:string)
            n115 = call <vilib>:"Add State(s) to Queue__jki_lib_state_machine.vi"("State(s) in Front (\"\")"="PGSQL: Close\nData: Cleanup\nEvents: Unregister", "State(s) in (\"\")"="Process: Sync", "State(s) at Back (\"\")"="Exit") -> ("States Out"=w323:string)  [unwired: 12 in]
            n116 = call <vilib>:"Add State(s) to Queue__jki_lib_state_machine.vi"("State(s) in (\"\")"=w328, "State(s) at Back (\"\")"=w323) -> ("States Out"=w327:string)  [unwired: 13 in]
            n117 = call <vilib>:"Add State(s) to Queue__jki_lib_state_machine.vi"("State(s) in Front (\"\")"=w327, "State(s) in (\"\")"=w333) -> ("States Out"=w332:string)  [unwired: 13 in]
          }
          frame "---------- Process ----------" {
            # "Template Separator\n(You can make a copy of, or modify, this frame)"
            n118 = call <vilib>:"Add State(s) to Queue__jki_lib_state_machine.vi"("State(s) in (\"\")"=w338) -> ("States Out"=w337:string)  [unwired: 14 in]
          }
          frame "Process: Sync" {
            n119 = Unbundle By Name(w346) -> ("SelfRef"=w342:refnum<class "Logger.PGSQL.lvclass">)
            n120 = call <vilib>:"WaitOnProcessSync.vi"("error in (no error)"=w341, "SMO"=w342) -> ("error out"=w340:errorcluster, "Don't run?"=w345:bool)  [unwired: 7 in, 1 out]
            n121 = Select(t="Data: Cleanup\nEvents: Unregister\nExit", s=w345, f="") -> (s? t:f=w339:string)
            n122 = call <vilib>:"Add State(s) to Queue__jki_lib_state_machine.vi"("State(s) in Front (\"\")"=w339, "State(s) in (\"\")"=w349) -> ("States Out"=w348:string)  [unwired: 13 in]
          }
          frame "---------- Events ----------" {
            # "Template Separator\n(You can make a copy of, or modify, this frame)"
            n123 = call <vilib>:"Add State(s) to Queue__jki_lib_state_machine.vi"("State(s) in (\"\")"=w354) -> ("States Out"=w353:string)  [unwired: 14 in]
          }
          frame "Events: Register" {
            # "Expand to add\nmore events"
            n124 = Unbundle By Name(w365) -> ("SelfRef"=w362:refnum<class "Logger.PGSQL.lvclass">)
            n125 = call <vilib>:"GetProtectedEvents.vi"("SMO"=w362) -> ("error out"=w358:errorcluster, "SMO Protected Events"=w363:T7, "SMO out"=w357:refnum<class "Logger.PGSQL.lvclass">)  [unwired: 8 in]
            n126 = call "Logger.GetPrivateEvents.vi"("Logger"=w357) -> ("error out"=w355:errorcluster, "Private Events"=w356:T8)  [unwired: 8 in, 1 out]
            n127 = register-events(w363, w356) -> (reference out=w364:refnum<event-registration>, error out=w359:errorcluster)  [unwired: 2 in]
            n128 = Merge Errors(w355, w361, w359, w358) -> (w360:errorcluster)
            n129 = call <vilib>:"Add State(s) to Queue__jki_lib_state_machine.vi"("State(s) in (\"\")"=w367) -> ("States Out"=w366:string)  [unwired: 14 in]
          }
          frame "Events: Unregister" {
            n130 = Unregister For Events(event registration refnum=w370, error in=w369) -> (error out=w368:errorcluster)
            n131 = call <vilib>:"Clear Errors.vi"("error in (no error)"=w368) -> ()  [unwired: 5 in, 2 out]
            n132 = call <vilib>:"Add State(s) to Queue__jki_lib_state_machine.vi"("State(s) in (\"\")"=w373) -> ("States Out"=w372:string)  [unwired: 14 in]
          }
          frame "---------- PGSQL ----------" {
            n133 = call <vilib>:"Add State(s) to Queue__jki_lib_state_machine.vi"("State(s) in (\"\")"=w378) -> ("States Out"=w377:string)  [unwired: 14 in]
          }
          frame "PGSQL: Connect" {
            n134 = Unbundle By Name(w383) -> ("SelfRef"=w382:refnum<class "Logger.PGSQL.lvclass">)
            n135 = call "Logger.PGSQL.Connect.vi"("error in (no error)"=w380, "Logger.PGSQL in"=w382) -> ("error out"=w379:errorcluster, "Logger.PGSQL out"=w381:refnum<class "Logger.PGSQL.lvclass">)  [unwired: 8 in]
            n136 = Bundle By Name(cluster=w383, "SelfRef"=w381) -> (w384:T4)
            n137 = call <vilib>:"Add State(s) to Queue__jki_lib_state_machine.vi"("State(s) in (\"\")"=w387) -> ("States Out"=w386:string)  [unwired: 14 in]
          }
          frame "PGSQL: Write" {
            n138 = Unbundle By Name(w406) -> ("SelfRef"=w411:refnum<class "Logger.PGSQL.lvclass">, "address"=w403:string, "data in"=w391:variant, "timestamps"=w392:timestamp[], "Write Time"=w390:timestamp)
            n139 = Unbundle By Name(w411) -> ("status"=w393:T2)
            n140 = case shown="Default" w389 {
              tunnel: [w415 w437] -> w407
              tunnel: w404 -> [w414 w436]
              tunnel: w403 -> [w424 w435]
              tunnel: [w423 w434] -> w402
              tunnel: [w412 w432] -> w401
              tunnel: [w420 w431] -> w400
              tunnel: [w422 w430] -> w398
              tunnel: w392 -> [w416 w429]
              tunnel: w391 -> [w413 w428]
              tunnel: w390 -> [w423 w427]
              tunnel: w411 -> [w418 w426]
              tunnel: [w417 w425] -> w388
              frame "Multiline" {
                n141 = call "Logger.PGSQL.WriteMultiline.vi"("timestamps"=w416, "error in (no error)"=w414, "data in"=w413, "address"=w424, "Logger.PGSQL in"=w418) -> ("error out"=w415:errorcluster, "Wrote to DB?"=w412:bool, "Logger.PGSQL out"=w417:refnum<class "Logger.PGSQL.lvclass">)  [unwired: 4 in]
                n142 = Get Date/Time In Seconds() -> (seconds since 1Jan1904=w422:timestamp)
                n143 = Select(t="Write Succesful", s=w412, f="Write Failed") -> (s? t:f=w420:string)
              }
              frame Default {
                n144 = call "Write Or Not.vi"("Time"=w427, "data in"=w428) -> ("Write?"=w433:bool)  [unwired: 1 in]
                n145 = case shown="True" w433 {
                  tunnel: [w441 w454] -> w437
                  tunnel: w436 -> [w441 w445]
                  tunnel: w435 -> [_ w450]
                  tunnel: [TRUE ("Wrote to DB?") w444] -> w432
                  tunnel: w428 -> [_ w449]
                  tunnel: [w443 w448] -> w434
                  tunnel: w427 -> [w443 _]
                  tunnel: ["Write Not Attempted" w451] -> w431
                  tunnel: [w439 w448] -> w430
                  tunnel: w429 -> [_ _]
                  tunnel: w426 -> [w438 w447]
                  tunnel: [w438 w446] -> w425
                  frame False {
                    n146 = Get Date/Time In Seconds() -> (seconds since 1Jan1904=w439:timestamp)
                  }
                  frame True {
                    n147 = call "Logger.PGSQL.Write.vi"("error in (no error)"=w445, "data in"=w449, "address"=w450, "Logger.PGSQL in"=w447) -> ("error out"=w454:errorcluster, "Wrote to DB?"=w444:bool, "Logger.PGSQL out"=w446:refnum<class "Logger.PGSQL.lvclass">)  [unwired: 5 in]
                    n148 = Select(t="Write Succesful", s=w444, f="Write Failed") -> (s? t:f=w451:string)
                    n149 = Get Date/Time In Seconds() -> (seconds since 1Jan1904=w448:timestamp)
                  }
                }
              }
            }
            n150 = case shown="Default" w393 {
              tunnel: w401 -> [_ w458]
              tunnel: ["" ("t") w457] -> w396
              frame "unconfigured" {
              }
              frame Default {
                n151 = Select(t="", s=w458, f="PGSQL: Close\nPGSQL: Connect") -> (s? t:f=w457:string)
              }
            }
            n152 = Format Into String(w400, w398) -> (resulting string=w397:string)  [unwired: 3 in, 1 out]
            n153 = call <vilib>:"Build State String with Arguments__JKI_lib_State_Machine.vi"("Arguments (\"\")"=w397, "State"="UI: Update Status") -> ("State with Arguments"=w394:string)  [unwired: 4 in]
            n154 = Bundle By Name(cluster=w406, "SelfRef"=w388, "Write Time"=w402) -> (w405:T4)
            n155 = call <vilib>:"Add State(s) to Queue__jki_lib_state_machine.vi"("State(s) in Front (\"\")"=w394, "State(s) at Back (\"\")"=w396) -> ("States Out"=w395:string)  [unwired: 13 in]
            n156 = call <vilib>:"Add State(s) to Queue__jki_lib_state_machine.vi"("State(s) in Front (\"\")"=w395, "State(s) in (\"\")"=w410) -> ("States Out"=w409:string)  [unwired: 13 in]
          }
          frame "PGSQL: Read" {
            n157 = Unbundle By Name(w464) -> ("SelfRef"=w463:refnum<class "Logger.PGSQL.lvclass">, "address"=w460:string)
            n158 = call "Logger.PGSQL.Read.vi"("error in (no error)"=w462, "address"=w460, "Logger.PGSQL in"=w463) -> ("error out"=w461:errorcluster)  [unwired: 8 in]
            n159 = call <vilib>:"Add State(s) to Queue__jki_lib_state_machine.vi"("State(s) in (\"\")"=w467) -> ("States Out"=w466:string)  [unwired: 14 in]
          }
          frame "PGSQL: Close" {
            n160 = Unbundle By Name(w473) -> ("SelfRef"=w470:refnum<class "Logger.PGSQL.lvclass">)
            n161 = call "Logger.PGSQL.Disconnect.vi"("error in (no error)"=w469, "Logger.PGSQL in"=w470) -> ("error out"=w468:errorcluster, "Logger.PGSQL out"=w471:refnum<class "Logger.PGSQL.lvclass">)  [unwired: 8 in]
            n162 = Bundle By Name(cluster=w473, "SelfRef"=w471) -> (w472:T4)
            n163 = call <vilib>:"Add State(s) to Queue__jki_lib_state_machine.vi"("State(s) in (\"\")"=w476) -> ("States Out"=w475:string)  [unwired: 14 in]
          }
        }
      }
    }
    frame Error {
    }
  }
  n164 = call-parent "Process.vi"("error in"=w5, "Logger"=w4) -> ("error out"=w3:errorcluster, "Logger out"=→"Logger out":refnum<class "Logger.PGSQL.lvclass">)  [unwired: 8 in]
  n165 = Merge Errors(w3, w2) -> (→"error out":errorcluster)
